vi "turnOnBECImageNaming.vi"(8 "error in (no error)":errorcluster, 10 "ImageRenaming":bool, 11 "CameraManager in":refnum<class "CameraManager.lvclass">) -> (0 "error out":errorcluster, 3 "CameraManager out":refnum<class "CameraManager.lvclass">)   [LabVIEW 2011, in "iManagement.lvlib" / "CameraManager.lvclass"]
doc: "Turn on BEC renaming, so that the pictures are named correctly after the acquisition"
uses:
  CameraManager.lvclass
  CameraManager.lvclass/CameraManager.ctl
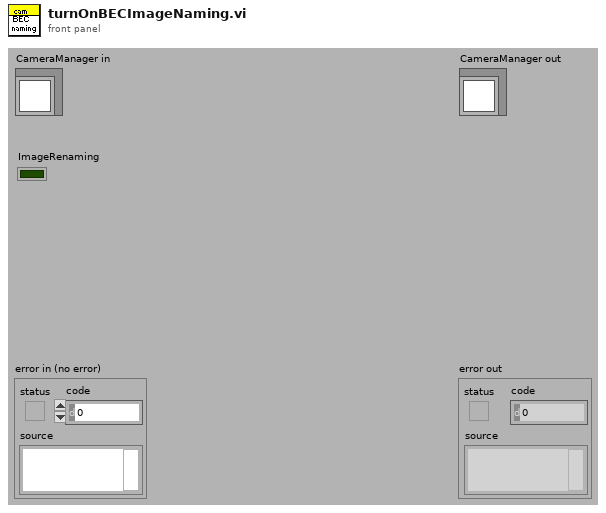
[diagram p1: front panel]
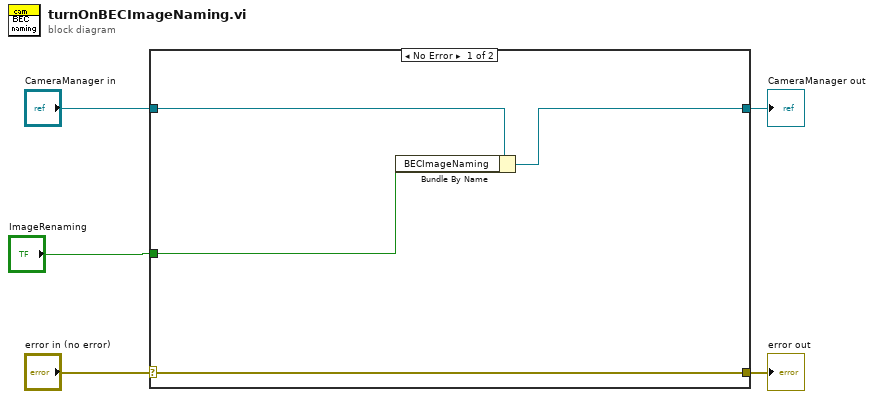
[diagram p0: block diagram]
diagram:
  n1 = case shown="No Error" "error in (no error)" {
    selector: "error in (no error)" -> [w9 w11]
    tunnel: [w9 w11] -> w4
    tunnel: [w7 w10] -> w2
    tunnel: "CameraManager in" -> [w8 w10]
    tunnel: "ImageRenaming" -> [w6 _]
    frame No Error {
      n2 = Bundle By Name(cluster=w8, "BECImageNaming"=w6) -> (w7:refnum<class "CameraManager.lvclass">)
    }
    frame Error {
    }
  }
  "error out" <- w4
  "CameraManager out" <- w2
